vi "Find Tracking Selection.vi"(0 "TrackingRowsUnits":i32[](array[numeric]), 7 "StateArray":i32[](array[numeric]), 11 "CurrentState":i32) -> (8 "TrackingRowsSel":i32[](array[numeric]))   [LabVIEW 2019]
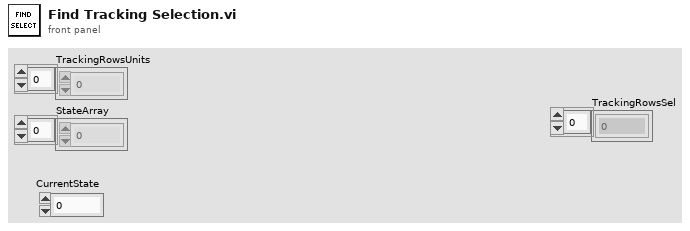
[diagram p1: front panel]
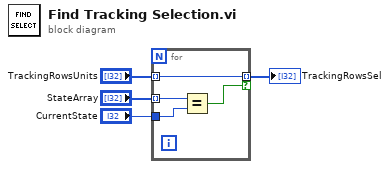
[diagram p0: block diagram]
diagram:
  n1 = for {
    tunnel: "StateArray" -> [w8] mode=indexing
    tunnel: "TrackingRowsUnits" -> [w6] mode=indexing
    tunnel: "CurrentState" -> [w7]
    tunnel: [w6] -> w1 mode=indexing if=w5
    n2 = Equal?(x=w8, y=w7) -> (x = y?=w5:bool)
  }
  "TrackingRowsSel" <- w1
